vi "rszvl_core_global.vi"() -> ()   [LabVIEW 2014] (continued)
"Repeated Capabilities"="", "Restricted Repeated Capabilities"="", "Help"="This attribute deletes the existing limit line and (re-)defines the physical units of the response values of the limit line.\n\nAvailable Repeated Capabilities:\nChannel: CH1,CH2,CH3,CH4,CH5,CH6,CH7,CH8,CH9,CH10,CH11,CH12,CH13,CH14,CH15,CH16,CH17,CH18,CH19,CH20\r\n\nRemote-control command(s):\nCALCulate<Chn>:LIMit:RDOMain:FORMat COMPlex | MAGNitude | PHASe | REAL | IMAGinary | SWR | GDELay | L | C", "Flags"={"OPC Wait"=FALSE, "Dont check status"=FALSE, "*WAI"=FALSE}, "Check Status Callback"=""}, {"Level"=2, "Descriptive Name"="NWA Limit Response Domain Spacing Units", "Class Only"=FALSE, "Data Type"=0, "Access"=1, "Identifier"="RSZVL_ATTR_NWA_LIMIT_RDOM_SPACING", "Range Table"="rszvl_rngNWALimitRDOMSpacing", "Command"="CALC{Channel}:LIM:RDOM:SPAC", "Read Callback"="", "Write Callback"="", "Range Callback"="", "Check Callback"="", "Rngtable Callback"="", "Coerce Callback"="", "User Callback"="", "Supported Models"="", "Instrument Options"="", "Repeated Capabilities"="", "Restricted Repeated Capabilities"="", "Help"="This attribute deletes the existing limit line and (re-)defines the physical units of the response values of the limit line.\n\nAvailable Repeated Capabilities:\nChannel: CH1,CH2,CH3,CH4,CH5,CH6,CH7,CH8,CH9,CH10,CH11,CH12,CH13,CH14,CH15,CH16,CH17,CH18,CH19,CH20\r\n\nRemote-control command(s):\nCALCulate<Chn>:LIMit:RDOMain:SPACing LINear | LOGarithmic | dB | SIC", "Flags"={"OPC Wait"=FALSE, "Dont check status"=FALSE, "*WAI"=FALSE}, "Check Status Callback"=""}, {"Level"=2, "Descriptive Name"="NWA Display Line State", "Class Only"=FALSE, "Data Type"=3, "Access"=2, "Identifier"="RSZVL_ATTR_NWA_DISPLAY_LINE_STATE", "Range Table"="", "Command"="CALC{Channel}:DLIN:STAT", "Read Callback"="", "Write Callback"="", "Range Callback"="", "Check Callback"="", "Rngtable Callback"="", "Coerce Callback"="", "User Callback"="", "Supported Models"="", "Instrument Options"="", "Repeated Capabilities"="", "Restricted Repeated Capabilities"="", "Help"="This attribute switches the horizontal line on or off.\n\nAvailable Repeated Capabilities:\nChannel: CH1,CH2,CH3,CH4,CH5,CH6,CH7,CH8,CH9,CH10,CH11,CH12,CH13,CH14,CH15,CH16,CH17,CH18,CH19,CH20\r\n\nRemote-control command(s):\nCALCulate<Chn>:DLINe:STATe ON | OFF", "Flags"={"OPC Wait"=FALSE, "Dont check status"=FALSE, "*WAI"=FALSE}, "Check Status Callback"=""}, {"Level"=2, "Descriptive Name"="NWA Display Line Position", "Class Only"=FALSE, "Data Type"=1, "Access"=2, "Identifier"="RSZVL_ATTR_NWA_DISPLAY_LINE_POSITION", "Range Table"="", "Command"="CALC{Channel}:DLIN", "Read Callback"="", "Write Callback"="", "Range Callback"="", "Check Callback"="", "Rngtable Callback"="", "Coerce Callback"="", "User Callback"="", "Supported Models"="", "Instrument Options"="", "Repeated Capabilities"="", "Restricted Repeated Capabilities"="", "Help"="This attribute defines the position (response value) of the horizontal line.\n\nAvailable Repeated Capabilities:\nChannel: CH1,CH2,CH3,CH4,CH5,CH6,CH7,CH8,CH9,CH10,CH11,CH12,CH13,CH14,CH15,CH16,CH17,CH18,CH19,CH20\r\n\nRemote-control command(s):\nCALCulate<Chn>:DLINe", "Flags"={"OPC Wait"=FALSE, "Dont check status"=FALSE, "*WAI"=FALSE}, "Check Status Callback"=""}, {"Level"=2, "Descriptive Name"="NWA Limit Segment Type", "Class Only"=FALSE, "Data Type"=0, "Access"=2, "Identifier"="RSZVL_ATTR_NWA_LIMIT_SEGM_TYPE", "Range Table"="rszvl_rngNWALimitSegmType", "Command"="CALC{Channel}:LIM:SEGM{Segment}:TYPE", "Read Callback"="", "Write Callback"="", "Range Callback"="", "Check Callback"="", "Rngtable Callback"="", "Coerce Callback"="", "User Callback"="", "Supported Models"="", "Instrument Options"="", "Repeated Capabilities"="", "Restricted Repeated Capabilities"="", "Help"="This attribute selects the limit line type for a limit line segment. This can be done before or after defining the stimulus and response values of the segment, however, a segment must be created first.\n\nAvailable Repeated Capabilities:\nChannel: CH1,CH2,CH3,CH4,CH5,CH6,CH7,CH8,CH9,CH10,CH11,CH12,CH13,CH14,CH15,CH16,CH17,CH18,CH19,CH20\r\nSegment: SEG1,SEG2,SEG3,SEG4,SEG5,SEG6,SEG7,SEG8,SEG9,SEG10,SEG11,SEG12,SEG13,SEG14,SEG15,SEG16,SEG17,SEG18,SEG19,SEG20\r\n\nRemote-control command(s):\nCALCulate<Chn>:LIMit:SEGMent<Seg>:TYPE LMIN | LMAX | OFF", "Flags"={"OPC Wait"=FALSE, "Dont check status"=FALSE, "*WAI"=FALSE}, "Check Status Callback"=""}, {"Level"=2, "Descriptive Name"="NWA Limit Segment Stimulus Start", "Class Only"=FALSE, "Data Type"=1, "Access"=2, "Identifier"="RSZVL_ATTR_NWA_LIMIT_SEGM_STIMUL_START", "Range Table"="", "Command"="CALC{Channel}:LIM:SEGM{Segment}:STIM:STAR", "Read Callback"="", "Write Callback"="", "Range Callback"="", "Check Callback"="", "Rngtable Callback"="", "Coerce Callback"="", "User Callback"="", "Supported Models"="", "Instrument Options"="", "Repeated Capabilities"="", "Restricted Repeated Capabilities"="", "Help"="This attribute changes the start stimulus value (i.e. the largest or smallest stimulus value) of a limit line segment. A segment must be created first.\n\nAvailable Repeated Capabilities:\nChannel: CH1,CH2,CH3,CH4,CH5,CH6,CH7,CH8,CH9,CH10,CH11,CH12,CH13,CH14,CH15,CH16,CH17,CH18,CH19,CH20\r\nSegment: SEG1,SEG2,SEG3,SEG4,SEG5,SEG6,SEG7,SEG8,SEG9,SEG10,SEG11,SEG12,SEG13,SEG14,SEG15,SEG16,SEG17,SEG18,SEG19,SEG20\r\n\nRemote-control command(s):\nCALCulate<Chn>:LIMit:SEGMent<Seg>:STIMulus:STARt", "Flags"={"OPC Wait"=FALSE, "Dont check status"=FALSE, "*WAI"=FALSE}, "Check Status Callback"=""}, {"Level"=2, "Descriptive Name"="NWa Limit Segment Stimulus Stop", "Class Only"=FALSE, "Data Type"=1, "Access"=2, "Identifier"="RSZVL_ATTR_NWA_LIMIT_SEGM_STIMUL_STOP", "Range Table"="", "Command"="CALC{Channel}:LIM:SEGM{Segment}:STIM:STOP", "Read Callback"="", "Write Callback"="", "Range Callback"="", "Check Callback"="", "Rngtable Callback"="", "Coerce Callback"="", "User Callback"="", "Supported Models"="", "Instrument Options"="", "Repeated Capabilities"="", "Restricted Repeated Capabilities"="", "Help"="This attribute changes the stop stimulus value (i.e. the largest or smallest stimulus value) of a limit line segment. A segment must be created first.\n\nAvailable Repeated Capabilities:\nChannel: CH1,CH2,CH3,CH4,CH5,CH6,CH7,CH8,CH9,CH10,CH11,CH12,CH13,CH14,CH15,CH16,CH17,CH18,CH19,CH20\r\nSegment: SEG1,SEG2,SEG3,SEG4,SEG5,SEG6,SEG7,SEG8,SEG9,SEG10,SEG11,SEG12,SEG13,SEG14,SEG15,SEG16,SEG17,SEG18,SEG19,SEG20\r\n\nRemote-control command(s):\nCALCulate<Chn>:LIMit:SEGMent<Seg>:STIMulus:STOP", "Flags"={"OPC Wait"=FALSE, "Dont check status"=FALSE, "*WAI"=FALSE}, "Check Status Callback"=""}, {"Level"=2, "Descriptive Name"="NWA Limit Segment Response Start", "Class Only"=FALSE, "Data Type"=1, "Access"=2, "Identifier"="RSZVL_ATTR_NWA_LIMIT_SEGM_RESPONSE_START", "Range Table"="", "Command"="CALC{Channel}:LIM:SEGM{Segment}:AMPL:STAR", "Read Callback"="", "Write Callback"="", "Range Callback"="", "Check Callback"="", "Rngtable Callback"="", "Coerce Callback"="", "User Callback"="", "Supported Models"="", "Instrument Options"="", "Repeated Capabilities"="", "Restricted Repeated Capabilities"="", "Help"="This attribute changes the start response value (i.e. the response value assigned to the start stimulus value) of a limit line segment. A segment must be created first.\n\nAvailable Repeated Capabilities:\nChannel: CH1,CH2,CH3,CH4,CH5,CH6,CH7,CH8,CH9,CH10,CH11,CH12,CH13,CH14,CH15,CH16,CH17,CH18,CH19,CH20\r\nSegment: SEG1,SEG2,SEG3,SEG4,SEG5,SEG6,SEG7,SEG8,SEG9,SEG10,SEG11,SEG12,SEG13,SEG14,SEG15,SEG16,SEG17,SEG18,SEG19,SEG20\r\n\nRemote-control command(s):\nCALCulate<Chn>:LIMit:SEGMent<Seg>:AMPLitude:STARt", "Flags"={"OPC Wait"=FALSE, "Dont check status"=FALSE, "*WAI"=FALSE}, "Check Status Callback"=""}, {"Level"=2, "Descriptive Name"="NWA Limit Segment Response Stop", "Class Only"=FALSE, "Data Type"=1, "Access"=2, "Identifier"="RSZVL_ATTR_NWA_LIMIT_SEGM_RESPONSE_STOP", "Range Table"="", "Command"="CALC{Channel}:LIM:SEGM{Segment}:AMPL:STOP", "Read Callback"="", "Write Callback"="", "Range Callback"="", "Check Callback"="", "Rngtable Callback"="", "Coerce Callback"="", "User Callback"="", "Supported Models"="", "Instrument Options"="", "Repeated Capabilities"="", "Restricted Repeated Capabilities"="", "Help"="This attribute changes the stop response value (i.e. the response value assigned to the stop stimulus value) of a limit line segment. A segment must be created first.\n\nAvailable Repeated Capabilities:\nChannel: CH1,CH2,CH3,CH4,CH5,CH6,CH7,CH8,CH9,CH10,CH11,CH12,CH13,CH14,CH15,CH16,CH17,CH18,CH19,CH20\r\nSegment: SEG1,SEG2,SEG3,SEG4,SEG5,SEG6,SEG7,SEG8,SEG9,SEG10,SEG11,SEG12,SEG13,SEG14,SEG15,SEG16,SEG17,SEG18,SEG19,SEG20\r\n\nRemote-control command(s):\nCALCulate<Chn>:LIMit:SEGMent<Seg>:AMPLitude:STOP", "Flags"={"OPC Wait"=FALSE, "Dont check status"=FALSE, "*WAI"=FALSE}, "Check Status Callback"=""}, {"Level"=2, "Descriptive Name"="NWA Limit Segment Stimulus Shift", "Class Only"=FALSE, "Data Type"=1, "Access"=1, "Identifier"="RSZVL_ATTR_NWA_LIMIT_SEGM_STIMUL_SHIFT", "Range Table"="", "Command"="CALC{Channel}:LIM:CONT:SHIF", "Read Callback"="", "Write Callback"="", "Range Callback"="", "Check Callback"="", "Rngtable Callback"="", "Coerce Callback"="", "User Callback"="", "Supported Models"="", "Instrument Options"="", "Repeated Capabilities"="", "Restricted Repeated Capabilities"="", "Help"="This attribute shifts the limit line in horizontal direction.\n\nAvailable Repeated Capabilities:\nChannel: CH1,CH2,CH3,CH4,CH5,CH6,CH7,CH8,CH9,CH10,CH11,CH12,CH13,CH14,CH15,CH16,CH17,CH18,CH19,CH20\r\n\nRemote-control command(s):\nCALCulate<Chn>:LIMit:CONTrol:SHIFt", "Flags"={"OPC Wait"=FALSE, "Dont check status"=FALSE, "*WAI"=FALSE}, "Check Status Callback"=""}, {"Level"=2, "Descriptive Name"="NWA Limit Segment Lower Shift", "Class Only"=FALSE, "Data Type"=1, "Access"=1, "Identifier"="RSZVL_ATTR_NWA_LIMIT_SEGM_LOWER_SHIFT", "Range Table"="", "Command"="CALC{Channel}:LIM:LOW:SHIF", "Read Callback"="", "Write Callback"="", "Range Callback"="", "Check Callback"="", "Rngtable Callback"="", "Coerce Callback"="", "User Callback"="", "Supported Models"="", "Instrument Options"="", "Repeated Capabilities"="", "Restricted Repeated Capabilities"="", "Help"="This attribute shifts all lower and upper limit line segments assigned to the active trace in vertical direction.\n\nAvailable Repeated Capabilities:\nChannel: CH1,CH2,CH3,CH4,CH5,CH6,CH7,CH8,CH9,CH10,CH11,CH12,CH13,CH14,CH15,CH16,CH17,CH18,CH19,CH20\r\n\nRemote-control command(s):\nCALCulate<Chn>:LIMit:LOWer:SHIFt", "Flags"={"OPC Wait"=FALSE, "Dont check status"=FALSE, "*WAI"=FALSE}, "Check Status Callback"=""}, {"Level"=2, "Descriptive Name"="NWA Limit Segment Upper Shift", "Class Only"=FALSE, "Data Type"=1, "Access"=1, "Identifier"="RSZVL_ATTR_NWA_LIMIT_SEGM_UPPER_SHIFT", "Range Table"="", "Command"="CALC{Channel}:LIM:UPP:SHIF", "Read Callback"="", "Write Callback"="", "Range Callback"="", "Check Callback"="", "Rngtable Callback"="", "Coerce Callback"="", "User Callback"="", "Supported Models"="", "Instrument Options"="", "Repeated Capabilities"="", "Restricted Repeated Capabilities"="", "Help"="This attribute shifts all lower and upper limit line segments assigned to the active trace in vertical direction.\n\nAvailable Repeated Capabilities:\nChannel: CH1,CH2,CH3,CH4,CH5,CH6,CH7,CH8,CH9,CH10,CH11,CH12,CH13,CH14,CH15,CH16,CH17,CH18,CH19,CH20\r\n\nRemote-control command(s):\nCALCulate<Chn>:LIMit:UPPer:SHIFt", "Flags"={"OPC Wait"=FALSE, "Dont check status"=FALSE, "*WAI"=FALSE}, "Check Status Callback"=""}, {"Level"=2, "Descriptive Name"="NWA Limit Segment Count", "Class Only"=FALSE, "Data Type"=0, "Access"=0, "Identifier"="RSZVL_ATTR_NWA_LIMIT_SEGM_COUNT", "Range Table"="", "Command"="CALC{Channel}:LIM:SEGM:COUN?", "Read Callback"="", "Write Callback"="", "Range Callback"="", "Check Callback"="", "Rngtable Callback"="", "Coerce Callback"="", "User Callback"="", "Supported Models"="", "Instrument Options"="", "Repeated Capabilities"="", "Restricted Repeated Capabilities"="", "Help"="This attribute queries the number of limit line segments.\n\nAvailable Repeated Capabilities:\nChannel: CH1,CH2,CH3,CH4,CH5,CH6,CH7,CH8,CH9,CH10,CH11,CH12,CH13,CH14,CH15,CH16,CH17,CH18,CH19,CH20\r\n\nRemote-control command(s):\nCALCulate<Chn>:LIMit:SEGMent<Seg>:COUNt?", "Flags"={"OPC Wait"=FALSE, "Dont check status"=FALSE, "*WAI"=FALSE}, "Check Status Callback"=""}, {"Level"=2, "Descriptive Name"="NWA Limit Delete All Segments", "Class Only"=FALSE, "Data Type"=4, "Access"=1, "Identifier"="RSZVL_ATTR_NWA_LIMIT_DELETE_ALL_SEGM", "Range Table"="", "Command"="CALC{Channel}:LIM:DEL:ALL", "Read Callback"="", "Write Callback"="", "Range Callback"="", "Check Callback"="", "Rngtable Callback"="", "Coerce Callback"="", "User Callback"="", "Supported Models"="", "Instrument Options"="", "Repeated Capabilities"="", "Restricted Repeated Capabilities"="", "Help"="This attribute deletes all limit line segments.\n\nAvailable Repeated Capabilities:\nChannel: CH1,CH2,CH3,CH4,CH5,CH6,CH7,CH8,CH9,CH10,CH11,CH12,CH13,CH14,CH15,CH16,CH17,CH18,CH19,CH20\r\n\nRemote-control command(s):\nCALCulate<Chn>:LIMit:DELete:ALL", "Flags"={"OPC Wait"=FALSE, "Dont check status"=FALSE, "*WAI"=FALSE}, "Check Status Callback"=""}, {"Level"=2, "Descriptive Name"="Ripple", "Class Only"=TRUE, "Data Type"=0, "Access"=0, "Identifier"="", "Range Table"="", "Command"="", "Read Callback"="", "Write Callback"="", "Range Callback"="", "Check Callback"="", "Rngtable Callback"="", "Coerce Callback"="", "User Callback"="", "Supported Models"="", "Instrument Options"="", "Repeated Capabilities"="", "Restricted Repeated Capabilities"="", "Help"="Put a help here", "Flags"={"OPC Wait"=FALSE, "Dont check status"=FALSE, "*WAI"=FALSE}, "Check Status Callback"=""}, {"Level"=3, "Descriptive Name"="NWA Ripple Check State", "Class Only"=FALSE, "Data Type"=3, "Access"=2, "Identifier"="RSZVL_ATTR_NWA_RIPPLE_CHECK_STATE", "Range Table"="", "Command"="CALC{Channel}:RIPP:STAT", "Read Callback"="", "Write Callback"="", "Range Callback"="", "Check Callback"="", "Rngtable Callback"="", "Coerce Callback"="", "User Callback"="", "Supported Models"="", "Instrument Options"="", "Repeated Capabilities"="", "Restricted Repeated Capabilities"="", "Help"="This attribute switches the global ripple limit check on or off. This check covers all traces in the active setup.\n\nAvailable Repeated Capabilities:\nChannel: CH1,CH2,CH3,CH4,CH5,CH6,CH7,CH8,CH9,CH10,CH11,CH12,CH13,CH14,CH15,CH16,CH17,CH18,CH19,CH20\r\n\nRemote-control command(s):\nCALCulate<Chn>:RIPPle:STATe ON | OFF", "Flags"={"OPC Wait"=FALSE, "Dont check status"=FALSE, "*WAI"=FALSE}, "Check Status Callback"=""}, {"Level"=3, "Descriptive Name"="NWA Get Ripple Global Limit Check Result", "Class Only"=FALSE, "Data Type"=0, "Access"=0, "Identifier"="RSZVL_ATTR_NWA_GET_RIPPLE_GLOBAL_LIMIT_CHECK_RESULT", "Range Table"="", "Command"="CALC{Channel}:RIPP:FAIL?", "Read Callback"="", "Write Callback"="", "Range Callback"="", "Check Callback"="", "Rngtable Callback"="", "Coerce Callback"="", "User Callback"="", "Supported Models"="", "Instrument Options"="", "Repeated Capabilities"="", "Restricted Repeated Capabilities"="", "Help"="This attribute returns a 0 or 1, to indicate whether or not the global ripple limit check has failed.\n\n0 represents pass (or a disabled limit check)\n1 represents fail in at least one ripple limit range\n\nAvailable Repeated Capabilities:\nChannel: CH1,CH2,CH3,CH4,CH5,CH6,CH7,CH8,CH9,CH10,CH11,CH12,CH13,CH14,CH15,CH16,CH17,CH18,CH19,CH20\r\n\nRemote-control command(s):\nCALCulate<Chn>:RIPPle:FAIL?", "Flags"={"OPC Wait"=FALSE, "Dont check status"=FALSE, "*WAI"=FALSE}, "Check Status Callback"=""}, {"Level"=3, "Descriptive Name"="NWA Ripple Range Segment Limit Check", "Class Only"=FALSE, "Data Type"=3, "Access"=2, "Identifier"="RSZVL_ATTR_NWA_RIPPLE_RANGE_SEGMENT_LIMIT_CHECK", "Range Table"="", "Command"="CALC{Channel}:RIPP:SEGM{Segment}:STAT", "Read Callback"="", "Write Callback"="", "Range Callback"="", "Check Callback"="", "Rngtable Callback"="", "Coerce Callback"="", "User Callback"="", "Supported Models"="", "Instrument Options"="", "Repeated Capabilities"="", "Restricted Repeated Capabilities"="", "Help"="This attribute enables or disables the limit check in the ripple limit range no. <Seg>.\n\nAvailable Repeated Capabilities:\nChannel: CH1,CH2,CH3,CH4,CH5,CH6,CH7,CH8,CH9,CH10,CH11,CH12,CH13,CH14,CH15,CH16,CH17,CH18,CH19,CH20\r\nSegment: SEG1,SEG2,SEG3,SEG4,SEG5,SEG6,SEG7,SEG8,SEG9,SEG10,SEG11,SEG12,SEG13,SEG14,SEG15,SEG16,SEG17,SEG18,SEG19,SEG20\r\n\nRemote-control command(s):\nCALCulate<Chn>:RIPPle:SEGMent<Seg>[:STATe] ON | OFF", "Flags"={"OPC Wait"=FALSE, "Dont check status"=FALSE, "*WAI"=FALSE}, "Check Status Callback"=""}, {"Level"=3, "Descriptive Name"="NWA Ripple Show Limits", "Class Only"=FALSE, "Data Type"=3, "Access"=2, "Identifier"="RSZVL_ATTR_NWA_RIPPLE_SHOW_LIMITS", "Range Table"="", "Command"="CALC{Channel}:RIPP:DISPlay:STAT", "Read Callback"="", "Write Callback"="", "Range Callback"="", "Check Callback"="", "Rngtable Callback"="", "Coerce Callback"="", "User Callback"="", "Supported Models"="", "Instrument Options"="", "Repeated Capabilities"="", "Restricted Repeated Capabilities"="", "Help"="This attribute displays or hides all ripple limit lines (including all ranges) associated to the active trace.\n\nAvailable Repeated Capabilities:\nChannel: CH1,CH2,CH3,CH4,CH5,CH6,CH7,CH8,CH9,CH10,CH11,CH12,CH13,CH14,CH15,CH16,CH17,CH18,CH19,CH20\r\n\nRemote-control command(s):\nCALCulate<Chn>:RIPPle:DISPlay[:STATe] ON | OFF", "Flags"={"OPC Wait"=FALSE, "Dont check status"=FALSE, "*WAI"=FALSE}, "Check Status Callback"=""}, {"Level"=3, "Descriptive Name"="NWA Ripple Range Segment Start", "Class Only"=FALSE, "Data Type"=1, "Access"=2, "Identifier"="RSZVL_ATTR_NWA_RIPPLE_RANGE_SEGMENT_START", "Range Table"="", "Command"="CALC{Channel}:RIPP:SEGM{Segment}:STIM:STAR", "Read Callback"="", "Write Callback"="", "Range Callback"="", "Check Callback"="", "Rngtable Callback"="", "Coerce Callback"="", "User Callback"="", "Supported Models"="", "Instrument Options"="", "Repeated Capabilities"="", "Restricted Repeated Capabilities"="", "Help"="This attribute changes the start stimulus value (i.e. the smallest stimulus value) of a ripple limit range. A range must be created first to enable this command (e.g CALCulate<Chn>:RIPPle:DATA).\n\nAvailable Repeated Capabilities:\nChannel: CH1,CH2,CH3,CH4,CH5,CH6,CH7,CH8,CH9,CH10,CH11,CH12,CH13,CH14,CH15,CH16,CH17,CH18,CH19,CH20\r\nSegment: SEG1,SEG2,SEG3,SEG4,SEG5,SEG6,SEG7,SEG8,SEG9,SEG10,SEG11,SEG12,SEG13,SEG14,SEG15,SEG16,SEG17,SEG18,SEG19,SEG20\r\n\nRemote-control command(s):\nCALCulate<Chn>:RIPPle:SEGMent<Seg>:STIMulus:STARt", "Flags"={"OPC Wait"=FALSE, "Dont check status"=FALSE, "*WAI"=FALSE}, "Check Status Callback"=""}, {"Level"=3, "Descriptive Name"="NWA Ripple Range Segment Stop", "Class Only"=FALSE, "Data Type"=1, "Access"=2, "Identifier"="RSZVL_ATTR_NWA_RIPPLE_RANGE_SEGMENT_STOP", "Range Table"="", "Command"="CALC{Channel}:RIPP:SEGM{Segment}:STIM:STOP", "Read Callback"="", "Write Callback"="", "Range Callback"="", "Check Callback"="", "Rngtable Callback"="", "Coerce Callback"="", "User Callback"="", "Supported Models"="", "Instrument Options"="", "Repeated Capabilities"="", "Restricted Repeated Capabilities"="", "Help"="This attribute changes the start stimulus value (i.e. the smallest stimulus value) of a ripple limit range. A range must be created first to enable this command (e.g CALCulate<Chn>:RIPPle:DATA).\n\nAvailable Repeated Capabilities:\nChannel: CH1,CH2,CH3,CH4,CH5,CH6,CH7,CH8,CH9,CH10,CH11,CH12,CH13,CH14,CH15,CH16,CH17,CH18,CH19,CH20\r\nSegment: SEG1,SEG2,SEG3,SEG4,SEG5,SEG6,SEG7,SEG8,SEG9,SEG10,SEG11,SEG12,SEG13,SEG14,SEG15,SEG16,SEG17,SEG18,SEG19,SEG20\r\n\nRemote-control command(s):\nCALCulate<Chn>:RIPPle:SEGMent<Seg>:STIMulus:STOP", "Flags"={"OPC Wait"=FALSE, "Dont check status"=FALSE, "*WAI"=FALSE}, "Check Status Callback"=""}, {"Level"=3, "Descriptive Name"="NWA Ripple Delete All Limit Ranges", "Class Only"=FALSE, "Data Type"=4, "Access"=1, "Identifier"="RSZVL_ATTR_NWA_RIPPLE_DELETE_ALL_LIMIT_RANGES", "Range Table"="", "Command"="CALC{Channel}:RIPP:DEL:ALL", "Read Callback"="", "Write Callback"="", "Range Callback"="", "Check Callback"="", "Rngtable Callback"="", "Coerce Callback"="", "User Callback"="", "Supported Models"="", "Instrument Options"="", "Repeated Capabilities"="", "Restricted Repeated Capabilities"="", "Help"="This attribute deletes all ripple limit ranges.\n\nAvailable Repeated Capabilities:\nChannel: CH1,CH2,CH3,CH4,CH5,CH6,CH7,CH8,CH9,CH10,CH11,CH12,CH13,CH14,CH15,CH16,CH17,CH18,CH19,CH20\r\n\nRemote-control command(s):\nCALCulate<Chn>:RIPPle:DELete:ALL", "Flags"={"OPC Wait"=FALSE, "Dont check status"=FALSE, "*WAI"=FALSE}, "Check Status Callback"=""}, {"Level"=3, "Descriptive Name"="NWA Ripple Limit Physical Units", "Class Only"=FALSE, "Data Type"=0, "Access"=1, "Identifier"="RSZVL_ATTR_NWA_RIPPLE_LIMIT_PHYSICAL_UNITS", "Range Table"="rszvl_rngRipplePhysicalUnits", "Command"="CALC{Channel}:RIPP:CONT:DOM", "Read Callback"="", "Write Callback"="", "Range Callback"="", "Check Callback"="", "Rngtable Callback"="", "Coerce Callback"="", "User Callback"="", "Supported Models"="", "Instrument Options"="", "Repeated Capabilities"="", "Restricted Repeated Capabilities"="", "Help"="This attribute deletes the existing ripple limit ranges and (re-)defines the physical units of the stimulus values of the ripple limit lines. The unit of the ripple limit is defined via CALCulate<Chn>:RIPPle:RDOMain:FORMat \n\nNotes:\n\n(1) The selected unit must be compatible with the sweep type ([SENSe<Ch>:]SWEep:TYPE); otherwise the limit line can not be displayed and no limit check is possible.\n\n(2) FLIN, FLOG, FSEG, and FSINgle select frequency units [default: Hz] for the limit line. \n\n(3) TLIN and TLOG select time units [default: s].\n\n(4) PLIN, PLOG and PSINgle select power units [default: dBm].\n\nAvailable Repeated Capabilities:\nChannel: CH1,CH2,CH3,CH4,CH5,CH6,CH7,CH8,CH9,CH10,CH11,CH12,CH13,CH14,CH15,CH16,CH17,CH18,CH19,CH20\r\n\nRemote-control command(s):\nCALCulate<Chn>:RIPPle:CONTrol:DOMain FLIN | FLOG | FSEG | FSINgle | TLIN | TLOG | PLIN | PLOG | PSINgle", "Flags"={"OPC Wait"=FALSE, "Dont check status"=FALSE, "*WAI"=FALSE}, "Check Status Callback"=""}, {"Level"=3, "Descriptive Name"="NWA Ripple Limit Response Domain Format Units", "Class Only"=FALSE, "Data Type"=0, "Access"=1, "Identifier"="RSZVL_ATTR_NWA_RIPPLE_LIMIT_RESPONSE_DOMAIN_FORMAT_UNITS", "Range Table"="rszvl_rngRippleFormUnits", "Command"="CALC{Channel}:RIPP:RDOM:FORM", "Read Callback"="", "Write Callback"="", "Range Callback"="", "Check Callback"="", "Rngtable Callback"="", "Coerce Callback"="", "User Callback"="", "Supported Models"="", "Instrument Options"="", "Repeated Capabilities"="", "Restricted Repeated Capabilities"="", "Help"="This attribute deletes the existing ripple limit ranges and (re-)defines the physical unit of the ripple limit. The units of the stimulus values are defined via CALCulate<Chn>:RIPPle:CONTrol:DOMain.\n\nNotes:\n\n(1) COMPlex, REAL, IMAGinary, and SWR select dimensionless numbers (U) for the limit line. \n\n(2) MAGNitude selects relative units (dB). \n\n(3) PHASe selects phase units (deg). \n\n(4) GDELay selects time units (s). \n\n(5) L selects inductance units (H/Henry). \n\n(6) C selects capacitance units (F/Farad).\n\nAvailable Repeated Capabilities:\nChannel: CH1,CH2,CH3,CH4,CH5,CH6,CH7,CH8,CH9,CH10,CH11,CH12,CH13,CH14,CH15,CH16,CH17,CH18,CH19,CH20\r\n\nRemote-control command(s):\nCALCulate<Chn>:RIPPle:RDOMain:FORMat COMPlex | MAGNitude | PHASe | REAL | IMAGinary | SWR | GDELay | L | C", "Flags"={"OPC Wait"=FALSE, "Dont check status"=FALSE, "*WAI"=FALSE}, "Check Status Callback"=""}, {"Level"=3, "Descriptive Name"="NWA Ripple Get Limit Ranges", "Class Only"=FALSE, "Data Type"=0, "Access"=0, "Identifier"="RSZVL_ATTR_NWA_RIPPLE_GET_LIMIT_RANGES", "Range Table"="", "Command"="CALC{Channel}:RIPP:SEGM:COUN?", "Read Callback"="", "Write Callback"="", "Range Callback"="", "Check Callback"="", "Rngtable Callback"="", "Coerce Callback"="", "User Callback"="", "Supported Models"="", "Instrument Options"="", "Repeated Capabilities"="", "Restricted Repeated Capabilities"="", "Help"="This attribute queries the number of ripple limit ranges.\n\nAvailable Repeated Capabilities:\nChannel: CH1,CH2,CH3,CH4,CH5,CH6,CH7,CH8,CH9,CH10,CH11,CH12,CH13,CH14,CH15,CH16,CH17,CH18,CH19,CH20\r\n\nRemote-control command(s):\nCALCulate<Chn>:RIPPle:SEGMent<Seg>:COUNt?", "Flags"={"OPC Wait"=FALSE, "Dont check status"=FALSE, "*WAI"=FALSE}, "Check Status Callback"=""}, {"Level"=3, "Descriptive Name"="NWA Ripple Limit Range", "Class Only"=FALSE, "Data Type"=1, "Access"=2, "Identifier"="RSZVL_ATTR_NWA_RIPPLE_LIMIT_RANGE", "Range Table"="", "Command"="CALC{Channel}:RIPP:SEGM{Segment}:LIM", "Read Callback"="", "Write Callback"="", "Range Callback"="", "Check Callback"="", "Rngtable Callback"="", "Coerce Callback"="", "User Callback"="", "Supported Models"="", "Instrument Options"="", "Repeated Capabilities"="", "Restricted Repeated Capabilities"="", "Help"="This attribute defines the ripple limit for ripple limit range no. <Seg>. A range must be created first to enable this command (e.g CALCulate<Chn>:RIPPle:DATA).\n\nAvailable Repeated Capabilities:\nChannel: CH1,CH2,CH3,CH4,CH5,CH6,CH7,CH8,CH9,CH10,CH11,CH12,CH13,CH14,CH15,CH16,CH17,CH18,CH19,CH20\r\nSegment: SEG1,SEG2,SEG3,SEG4,SEG5,SEG6,SEG7,SEG8,SEG9,SEG10,SEG11,SEG12,SEG13,SEG14,SEG15,SEG16,SEG17,SEG18,SEG19,SEG20\r\n\nRemote-control command(s):\nCALCulate<Chn>:RIPPle:SEGMent<Seg>:LIMit", "Flags"={"OPC Wait"=FALSE, "Dont check status"=FALSE, "*WAI"=FALSE}, "Check Status Callback"=""}, {"Level"=1, "Descriptive Name"="NWA Measurement", "Class Only"=TRUE, "Data Type"=0, "Access"=0, "Identifier"="", "Range Table"="", "Command"="", "Read Callback"="", "Write Callback"="", "Range Callback"="", "Check Callback"="", "Rngtable Callback"="", "Coerce Callback"="", "User Callback"="", "Supported Models"="", "Instrument Options"="", "Repeated Capabilities"="", "Restricted Repeated Capabilities"="", "Help"="(1) NWA Get Limit Check Result:\nThis attribute returns a 0 or 1, to indicate whether or not the limit check has failed. \n\n(2) NWA Get Combined Limit Check Result:\nThis attribute returns a 0 or 1, to indicate whether or not a composite limit check on several traces has failed.\n\n(3) NWA Get Reference Marker Response:\nThis attribute returns the response (in Cartesian diagrams: y-axis) value of the reference marker. The reference marker must be created before using CALCulate<Chn>:MARKer<Mk>:REFerence[:STATe] ON.\n\n(4) NWA Marker Position:\nThis attribute defines the stimulus (in Cartesian diagrams: x-axis) value of the marker no. <Mk>, which can (but doesn't have to) be created using CALCulate<Chn>:MARKer<Mk>[:STATe] ON.\n\n(5) NWA Marker Amplitude:\nThis attribute returns the response (in Cartesian diagrams: y-axis) value of marker no. <Mk>. The marker must be created before using CALCulate<Chn>:MARKer<Mk>[:STATe] ON.\n\n(6) NWA Low-Level Measurement (Class):\nPut a help here\n\n(7) NWA Measurement Parameter (Class):\nPut a help here\n\n(8) NWA Distance To Fault (Class):\nPut a help here", "Flags"={"OPC Wait"=FALSE, "Dont check status"=FALSE, "*WAI"=FALSE}, "Check Status Callback"=""}, {"Level"=2, "Descriptive Name"="NWA Get Limit Check Result", "Class Only"=FALSE, "Data Type"=0, "Access"=0, "Identifier"="RSZVL_ATTR_NWA_LIMIT_CHECK_RESULT", "Range Table"="", "Command"="CALC{Channel}:LIM:FAIL?", "Read Callback"="", "Write Callback"="", "Range Callback"="", "Check Callback"="", "Rngtable Callback"="", "Coerce Callback"="", "User Callback"="", "Supported Models"="", "Instrument Options"="", "Repeated Capabilities"="", "Restricted Repeated Capabilities"="", "Help"="This attribute returns a 0 or 1, to indicate whether or not the limit check has failed.\n\nAvailable Repeated Capabilities:\nChannel: CH1,CH2,CH3,CH4,CH5,CH6,CH7,CH8,CH9,CH10,CH11,CH12,CH13,CH14,CH15,CH16,CH17,CH18,CH19,CH20\r\n\nRemote-control command(s):\nCALCulate<Chn>:LIMit:FAIL?", "Flags"={"OPC Wait"=FALSE, "Dont check status"=FALSE, "*WAI"=FALSE}, "Check Status Callback"=""}, {"Level"=2, "Descriptive Name"="NWA Get Combined Limit Check Result", "Class Only"=FALSE, "Data Type"=0, "Access"=0, "Identifier"="RSZVL_ATTR_NWA_CLIMIT_CHECK_RESULT", "Range Table"="", "Command"="CALC:CLIM:FAIL?", "Read Callback"="", "Write Callback"="", "Range Callback"="", "Check Callback"="", "Rngtable Callback"="", "Coerce Callback"="", "User Callback"="", "Supported Models"="", "Instrument Options"="", "Repeated Capabilities"="", "Restricted Repeated Capabilities"="", "Help"="This attribute returns a 0 or 1, to indicate whether or not a composite limit check on several traces has failed.\n\nAvailable Repeated Capabilities:\nNone\n\nRemote-control command(s):\nCALCulate<Chn>:CLIMits:FAIL?", "Flags"={"OPC Wait"=FALSE, "Dont check status"=FALSE, "*WAI"=FALSE}, "Check Status Callback"=""}, {"Level"=2, "Descriptive Name"="NWA Get Reference Marker Response", "Class Only"=FALSE, "Data Type"=1, "Access"=0, "Identifier"="RSZVL_ATTR_NWA_REFER_MARKER_RESPONSE", "Range Table"="", "Command"="CALC{Channel}:MARK:REF:Y?", "Read Callback"="", "Write Callback"="", "Range Callback"="", "Check Callback"="", "Rngtable Callback"="", "Coerce Callback"="", "User Callback"="", "Supported Models"="", "Instrument Options"="", "Repeated Capabilities"="", "Restricted Repeated Capabilities"="", "Help"="This attribute returns the response (in Cartesian diagrams: y-axis) value of the reference marker. The reference marker must be created before using CALCulate<Chn>:MARKer<Mk>:REFerence[:STATe] ON.\n\nAvailable Repeated Capabilities:\nChannel: CH1,CH2,CH3,CH4,CH5,CH6,CH7,CH8,CH9,CH10,CH11,CH12,CH13,CH14,CH15,CH16,CH17,CH18,CH19,CH20\r\n\nRemote-control command(s):\nCALCulate<Chn>:MARKer<Mk>:REFerence:Y?", "Flags"={"OPC Wait"=FALSE, "Dont check status"=FALSE, "*WAI"=FALSE}, "Check Status Callback"=""}, {"Level"=2, "Descriptive Name"="NWA Marker Position", "Class Only"=FALSE, "Data Type"=1, "Access"=2, "Identifier"="RSZVL_ATTR_NWA_MARKER_POSITION", "Range Table"="", "Command"="CALC{Channel}:MARK{NWAMarker}:X", "Read Callback"="", "Write Callback"="", "Range Callback"="", "Check Callback"="", "Rngtable Callback"="", "Coerce Callback"="", "User Callback"="", "Supported Models"="", "Instrument Options"="", "Repeated Capabilities"="", "Restricted Repeated Capabilities"="", "Help"="This attribute defines the stimulus (in Cartesian diagrams: x-axis) value of the marker no. <Mk>, which can (but doesn't have to) be created using CALCulate<Chn>:MARKer<Mk>[:STATe] ON.\n\nAvailable Repeated Capabilities:\nChannel: CH1,CH2,CH3,CH4,CH5,CH6,CH7,CH8,CH9,CH10,CH11,CH12,CH13,CH14,CH15,CH16,CH17,CH18,CH19,CH20\r\nNWAMarker: MAR1,MAR2,MAR3,MAR4,MAR5,MAR6,MAR7,MAR8,MAR9,MAR10\r\n\nRemote-control command(s):\nCALCulate<Chn>:MARKer<Mk>:X", "Flags"={"OPC Wait"=FALSE, "Dont check status"=FALSE, "*WAI"=FALSE}, "Check Status Callback"=""}, {"Level"=2, "Descriptive Name"="NWA Marker Amplitude", "Class Only"=FALSE, "Data Type"=1, "Access"=0, "Identifier"="RSZVL_ATTR_NWA_MARKER_AMPLITUDE", "Range Table"="", "Command"="CALC{Channel}:MARK{NWAMarker}:Y?", "Read Callback"="", "Write Callback"="", "Range Callback"="", "Check Callback"="", "Rngtable Callback"="", "Coerce Callback"="", "User Callback"="", "Supported Models"="", "Instrument Options"="", "Repeated Capabilities"="", "Restricted Repeated Capabilities"="", "Help"="This attribute returns the response (in Cartesian diagrams: y-axis) value of marker no. <Mk>. The marker must be created before using CALCulate<Chn>:MARKer<Mk>[:STATe] ON.\n\nAvailable Repeated Capabilities:\nChannel: CH1,CH2,CH3,CH4,CH5,CH6,CH7,CH8,CH9,CH10,CH11,CH12,CH13,CH14,CH15,CH16,CH17,CH18,CH19,CH20\r\nNWAMarker: MAR1,MAR2,MAR3,MAR4,MAR5,MAR6,MAR7,MAR8,MAR9,MAR10\r\n\nRemote-control command(s):\nCALCulate<Chn>:MARKer<Mk>:Y?", "Flags"={"OPC Wait"=FALSE, "Dont check status"=FALSE, "*WAI"=FALSE}, "Check Status Callback"=""}, {"Level"=2, "Descriptive Name"="NWA Low-Level Measurement", "Class Only"=TRUE, "Data Type"=0, "Access"=0, "Identifier"="", "Range Table"="", "Command"="", "Read Callback"="", "Write Callback"="", "Range Callback"="", "Check Callback"="", "Rngtable Callback"="", "Coerce Callback"="", "User Callback"="", "Supported Models"="", "Instrument Options"="", "Repeated Capabilities"="", "Restricted Repeated Capabilities"="", "Help"="Put a help here", "Flags"={"OPC Wait"=FALSE, "Dont check status"=FALSE, "*WAI"=FALSE}, "Check Status Callback"=""}, {"Level"=3, "Descriptive Name"="NWA Initiate", "Class Only"=FALSE, "Data Type"=4, "Access"=1, "Identifier"="RSZVL_ATTR_NWA_INIT", "Range Table"="", "Command"="INIT{Channel}:IMM", "Read Callback"="", "Write Callback"="", "Range Callback"="", "Check Callback"="", "Rngtable Callback"="", "Coerce Callback"="", "User Callback"="", "Supported Models"="", "Instrument Options"="", "Repeated Capabilities"="", "Restricted Repeated Capabilities"="", "Help"="This attribute starts a new single sweep sequence. This command is available in single sweep mode only (INITiate<Ch>:CONTinuous OFF).\n\nAvailable Repeated Capabilities:\nChannel: CH1,CH2,CH3,CH4,CH5,CH6,CH7,CH8,CH9,CH10,CH11,CH12,CH13,CH14,CH15,CH16,CH17,CH18,CH19,CH20\r\n\nRemote-control command(s):\nINITiate<Ch>[:IMMediate]", "Flags"={"OPC Wait"=TRUE, "Dont check status"=FALSE, "*WAI"=FALSE}, "Check Status Callback"=""}, {"Level"=2, "Descriptive Name"="NWA Measurement Parameter", "Class Only"=TRUE, "Data Type"=0, "Access"=0, "Identifier"="", "Range Table"="", "Command"="", "Read Callback"="", "Write Callback"="", "Range Callback"="", "Check Callback"="", "Rngtable Callback"="", "Coerce Callback"="", "User Callback"="", "Supported Models"="", "Instrument Options"="", "Repeated Capabilities"="", "Restricted Repeated Capabilities"="", "Help"="Put a help here", "Flags"={"OPC Wait"=FALSE, "Dont check status"=FALSE, "*WAI"=FALSE}, "Check Status Callback"=""}, {"Level"=3, "Descriptive Name"="NWA Parameter Conversion", "Class Only"=FALSE, "Data Type"=0, "Access"=2, "Identifier"="RSZVL_ATTR_NWA_PARAMETER_CONVERSION", "Range Table"="rszvl_rngNWAParamConversion", "Command"="CALC{Channel}:TRAN:COMP", "Read Callback"="", "Write Callback"="", "Range Callback"="", "Check Callback"="", "Rngtable Callback"="", "Coerce Callback"="", "User Callback"="", "Supported Models"="", "Instrument Options"="", "Repeated Capabilities"="", "Restricted Repeated Capabilities"="", "Help"="This attribute converts S-parameters into matched-circuit (converted) Y-parameters or Z-parameters and vice versa.\n\nAvailable Repeated Capabilities:\nChannel: CH1,CH2,CH3,CH4,CH5,CH6,CH7,CH8,CH9,CH10,CH11,CH12,CH13,CH14,CH15,CH16,CH17,CH18,CH19,CH20\r\n\nRemote-control command(s):\nCALCulate<Chn>:TRANsform:COMPlex S | Y | Z", "Flags"={"OPC Wait"=FALSE, "Dont check status"=FALSE, "*WAI"=FALSE}, "Check Status Callback"=""}, {"Level"=2, "Descriptive Name"="NWA Distance To Fault", "Class Only"=TRUE, "Data Type"=0, "Access"=0, "Identifier"="", "Range Table"="", "Command"="", "Read Callback"="", "Write Callback"="", "Range Callback"="", "Check Callback"="", "Rngtable Callback"="", "Coerce Callback"="", "User Callback"="", "Supported Models"="", "Instrument Options"="", "Repeated Capabilities"="", "Restricted Repeated Capabilities"="", "Help"="Put a help here", "Flags"={"OPC Wait"=FALSE, "Dont check status"=FALSE, "*WAI"=FALSE}, "Check Status Callback"=""}, {"Level"=3, "Descriptive Name"="NWA Distance To Fault State", "Class Only"=FALSE, "Data Type"=3, "Access"=2, "Identifier"="RSZVL_ATTR_NWA_DFAULT_STATE", "Range Table"="", "Command"="CALC{Channel}:TRAN:DTF:STAT", "Read Callback"="", "Write Callback"="", "Range Callback"="", "Check Callback"="", "Rngtable Callback"="", "Coerce Callback"="", "User Callback"="", "Supported Models"="", "Instrument Options"="", "Repeated Capabilities"="", "Restricted Repeated Capabilities"="", "Help"="This attribute enables or disables the distance-to-fault measurement.\n\nAvailable Repeated Capabilities:\nChannel: CH1,CH2,CH3,CH4,CH5,CH6,CH7,CH8,CH9,CH10,CH11,CH12,CH13,CH14,CH15,CH16,CH17,CH18,CH19,CH20\r\n\nRemote-control command(s):\nCALCulate<Chn>:TRANsform:DTFault:STATe ON | OFF", "Flags"={"OPC Wait"=FALSE, "Dont check status"=FALSE, "*WAI"=FALSE}, "Check Status Callback"=""}, {"Level"=3, "Descriptive Name"="NWA Distance To Fault Start Distance", "Class Only"=FALSE, "Data Type"=1, "Access"=2, "Identifier"="RSZVL_ATTR_NWA_DFAULT_START", "Range Table"="rszvl_rngNWADFaultStart", "Command"="CALC{Channel}:TRAN:DTF:STAR", "Read Callback"="", "Write Callback"="", "Range Callback"="", "Check Callback"="", "Rngtable Callback"="", "Coerce Callback"="", "User Callback"="", "Supported Models"="", "Instrument Options"="", "Repeated Capabilities"="", "Restricted Repeated Capabilities"="", "Help"="This attribute defines the start distance of the distance-to-fault diagram.\n\nAvailable Repeated Capabilities:\nChannel: CH1,CH2,CH3,CH4,CH5,CH6,CH7,CH8,CH9,CH10,CH11,CH12,CH13,CH14,CH15,CH16,CH17,CH18,CH19,CH20\r\n\nRemote-control command(s):\nCALCulate<Chn>:TRANsform:DTFault:STARt", "Flags"={"OPC Wait"=FALSE, "Dont check status"=FALSE, "*WAI"=FALSE}, "Check Status Callback"=""}, {"Level"=3, "Descriptive Name"="NWA Distance To Fault Stop Distance", "Class Only"=FALSE, "Data Type"=1, "Access"=2, "Identifier"="RSZVL_ATTR_NWA_DFAULT_STOP", "Range Table"="rszvl_rngNWADFaultStop", "Command"="CALC{Channel}:TRAN:DTF:STOP", "Read Callback"="", "Write Callback"="", "Range Callback"="", "Check Callback"="", "Rngtable Callback"="", "Coerce Callback"="", "User Callback"="", "Supported Models"="", "Instrument Options"="", "Repeated Capabilities"="", "Restricted Repeated Capabilities"="", "Help"="This attribute defines the stop distance of the distance-to-fault diagram.\n\nAvailable Repeated Capabilities:\nChannel: CH1,CH2,CH3,CH4,CH5,CH6,CH7,CH8,CH9,CH10,CH11,CH12,CH13,CH14,CH15,CH16,CH17,CH18,CH19,CH20\r\n\nRemote-control command(s):\nCALCulate<Chn>:TRANsform:DTFault:STOP", "Flags"={"OPC Wait"=FALSE, "Dont check status"=FALSE, "*WAI"=FALSE}, "Check Status Callback"=""}, {"Level"=3, "Descriptive Name"="NWA Distance To Fault Center Distance", "Class Only"=FALSE, "Data Type"=1, "Access"=2, "Identifier"="RSZVL_ATTR_NWA_DFAULT_CENTER", "Range Table"="rszvl_rngNWADFaultStop", "Command"="CALC{Channel}:TRAN:DTF:CENT", "Read Callback"="", "Write Callback"="", "Range Callback"="", "Check Callback"="", "Rngtable Callback"="", "Coerce Callback"="", "User Callback"="", "Supported Models"="", "Instrument Options"="", "Repeated Capabilities"="", "Restricted Repeated Capabilities"="", "Help"="This attribute defines the center distance of the distance-to-fault diagram.\n\nAvailable Repeated Capabilities:\nChannel: CH1,CH2,CH3,CH4,CH5,CH6,CH7,CH8,CH9,CH10,CH11,CH12,CH13,CH14,CH15,CH16,CH17,CH18,CH19,CH20\r\n\nRemote-control command(s):\nCALCulate<Chn>:TRANsform:DTFault:CENTer", "Flags"={"OPC Wait"=FALSE, "Dont check status"=FALSE, "*WAI"=FALSE}, "Check Status Callback"=""}, {"Level"=3, "Descriptive Name"="NWA Distance To Fault Span", "Class Only"=FALSE, "Data Type"=1, "Access"=2, "Identifier"="RSZVL_ATTR_NWA_DFAULT_SPAN", "Range Table"="rszvl_rngNWADFaultSpan", "Command"="CALC{Channel}:TRAN:DTF:SPAN", "Read Callback"="", "Write Callback"="", "Range Callback"="", "Check Callback"="", "Rngtable Callback"="", "Coerce Callback"="", "User Callback"="", "Supported Models"="", "Instrument Options"="", "Repeated Capabilities"="", "Restricted Repeated Capabilities"="", "Help"="This attribute defines the span of the distance-to-fault diagram.\n\nAvailable Repeated Capabilities:\nChannel: CH1,CH2,CH3,CH4,CH5,CH6,CH7,CH8,CH9,CH10,CH11,CH12,CH13,CH14,CH15,CH16,CH17,CH18,CH19,CH20\r\n\nRemote-control command(s):\nCALCulate<Chn>:TRANsform:DTFault:SPAN", "Flags"={"OPC Wait"=FALSE, "Dont check status"=FALSE, 
